vi "ErrorCheckCRC.vi"(8 "error in (no error)":errorcluster, 11 "Message w CRC":u8[](array[numeric]) format="%.0x") -> (0 "error out":errorcluster, 3 "Message w/ CRC":u8[](array[numeric]))   [LabVIEW 2015, in "navX Library v3.lvlib" / "navX - SPI.lvclass"]
uses:
  navX - SPI.lvclass
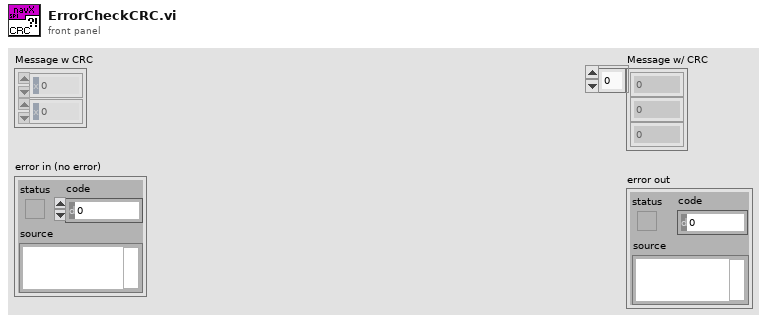
[diagram p1: front panel]
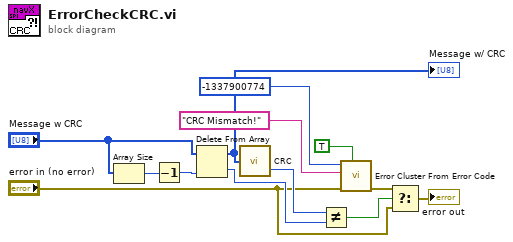
[diagram p0: block diagram]
diagram:
  n1 = Array Size(array="Message w CRC") -> (size(s)=w12:i32)
  n2 = Decrement(x=w12) -> (x-1=w1:i32)
  n3 = Delete From Array(array="Message w CRC", index=w1) -> (deleted portion=w8:u8, array with subset deleted=w2:u8[])  [unwired: 1 in]
  "Message w/ CRC" <- w2
  n4 = call "CRC.vi"("Message"=w2) -> ("CRC"=w7:u8)  [unwired: 1 out]
  n5 = Not Equal?(x=w7, y=w8) -> (x != y?=w3:bool)
  n6 = call <vilib>:"Error Cluster From Error Code.vi"("show call chain? (False)"=TRUE, "error in (no error)"="error in (no error)", "error message (\"\")"="CRC Mismatch!" ("error message (\"\")"), "error code (0)"=-1337900774) -> ("error out"=w6:errorcluster)  [unwired: 5 in]
  n7 = Select(t=w6, s=w3, f="error in (no error)") -> (s? t:f=→"error out":errorcluster)
